vi "Manual-Tester.vi"() -> ()   [LabVIEW 2017]
doc: "Use this template to build a producer/consumer design pattern with events to produce queue items. Use this design pattern instead of the User Interface Event Handler pattern for user interfaces when you want to execute code asynchronously in response to an event without slowing the user interface responsiveness."
uses:
  Events.ctl
  FpgaInterface/FpgaInterface.lvclass
panel:
  out "error out":errorcluster
  in  "error in (no error)":errorcluster
  in  "Write all GPIO":bool
  in  "GPIO #2":u32
  in  "GPIO #1":u32
  out "Elements Remaining":u32
  out "Payload 2":u8[](array[numeric])=[160, 32, 195, 223] format="%.0x"
  out "GPIO #2":u32
  out "GPIO #1":u32
  in  "Payload":u8[](array[numeric])=[160, 32, 195, 223] format="%.0x"
  in  "Read from FIFO #1":bool
  in  "Write to FIFO #1":bool
  out "Status":string
  in  "Read all GPIO":bool
  in  "stop":bool
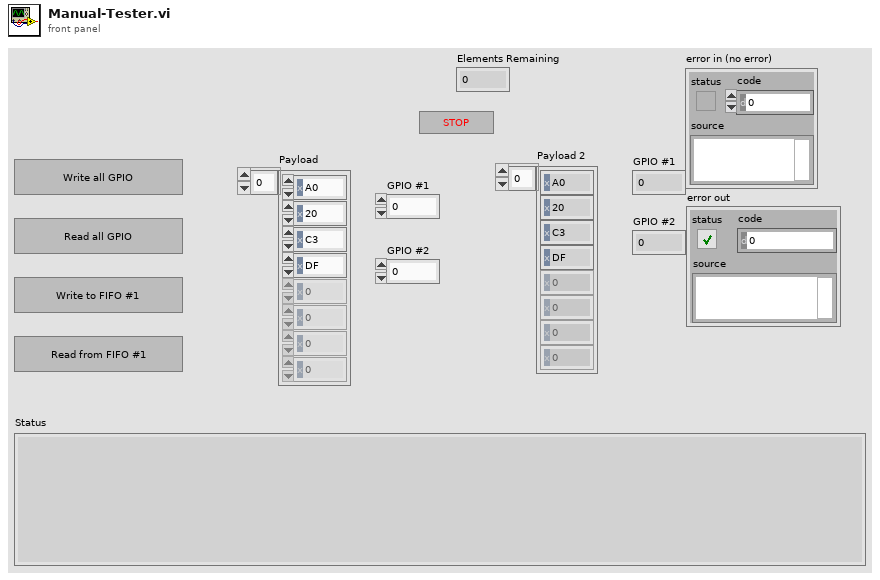
[diagram p1: front panel]
types:
  T1 = typedef "Events.ctl" = enum16{"Open FPGA", "Write to GPIO", "Read all GPIO", "Write to Fifo #1", "Read from Fifo #1", "Close FPGA"}
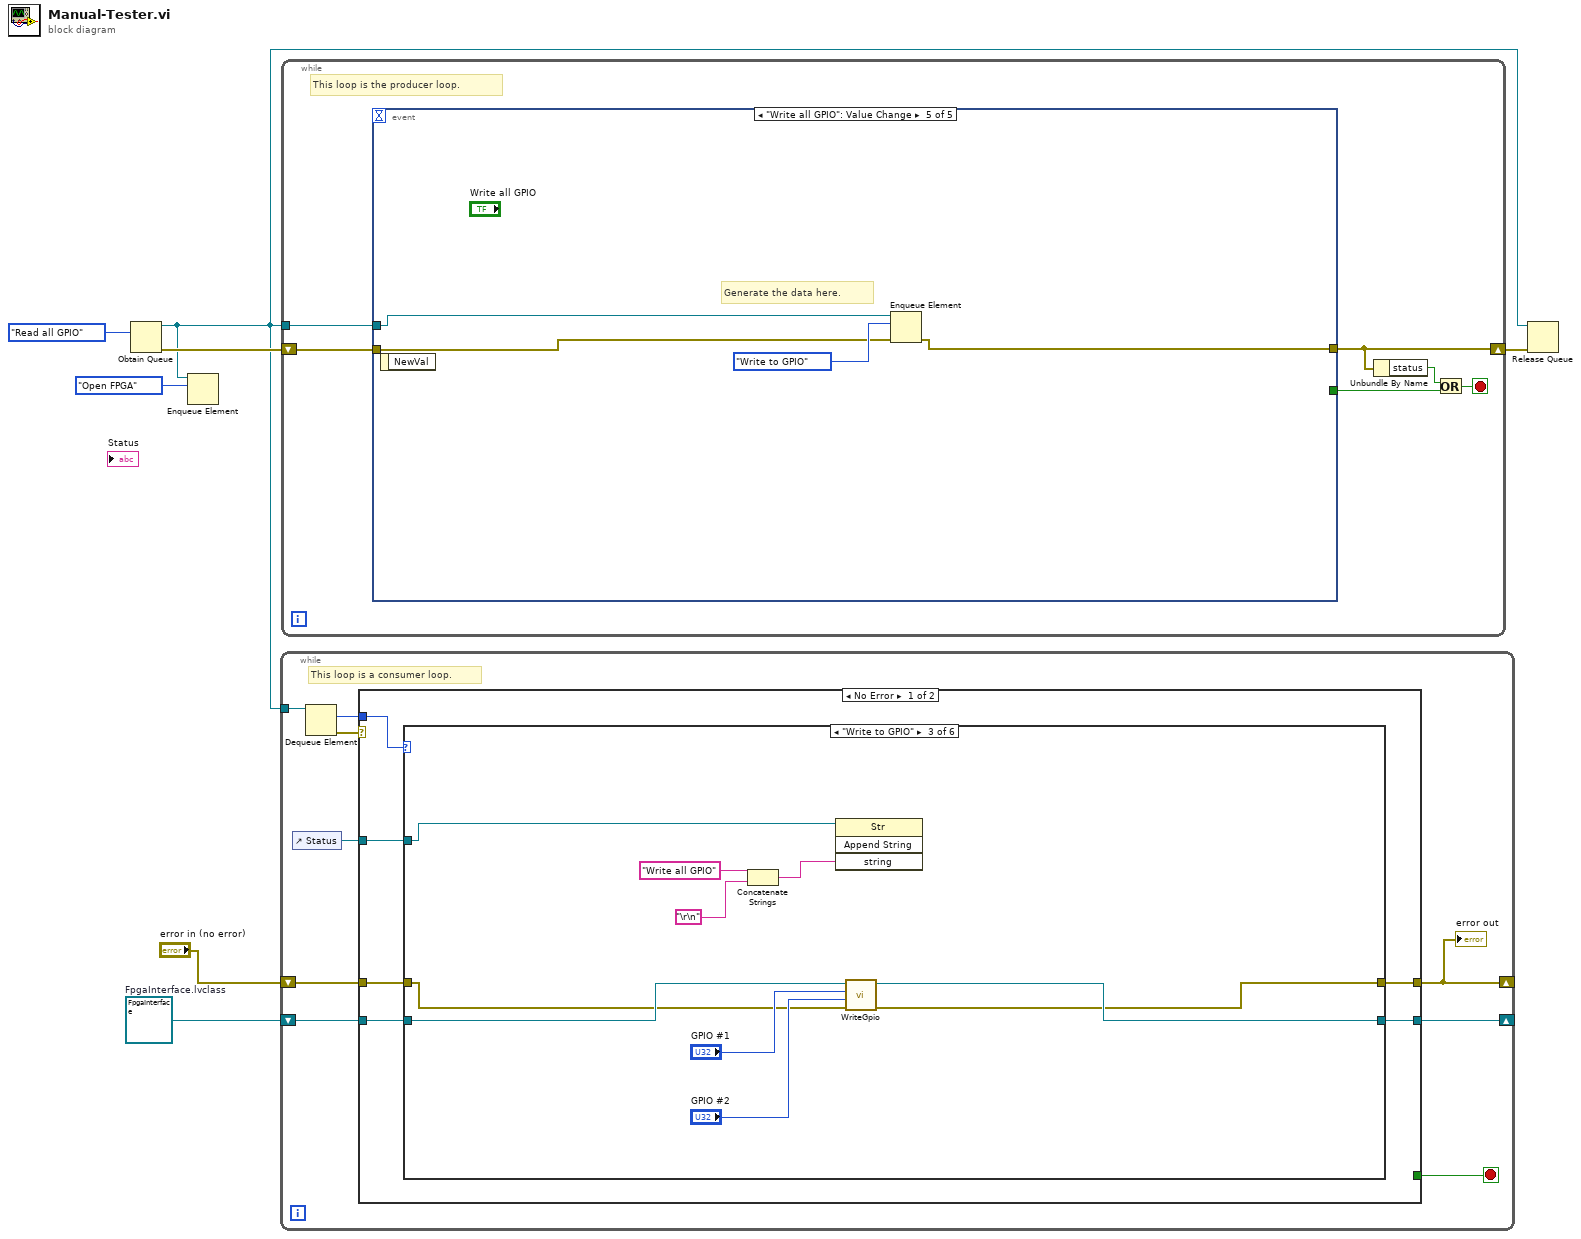
[diagram p0: block diagram]
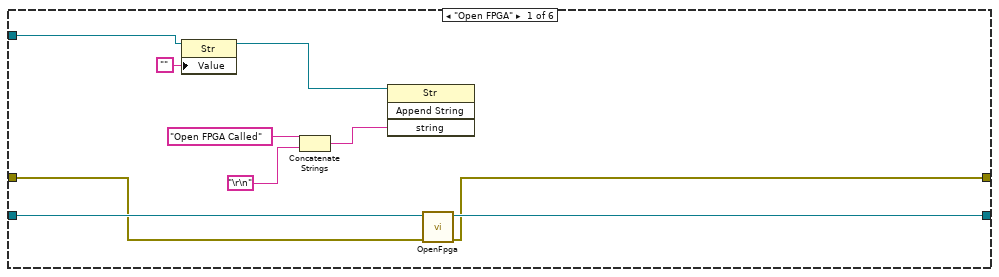
[diagram p2: hidden frame]
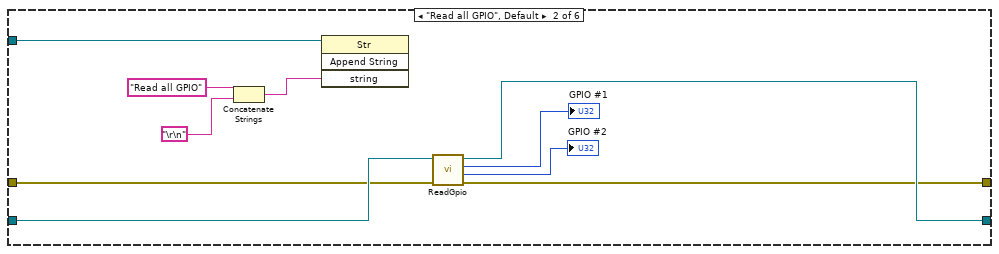
[diagram p3: hidden frame]
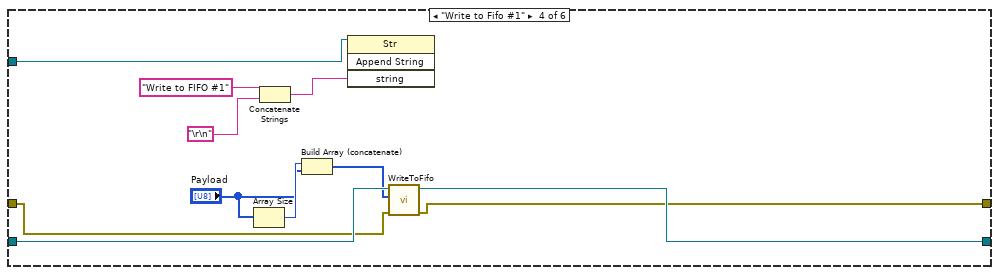
[diagram p4: hidden frame]
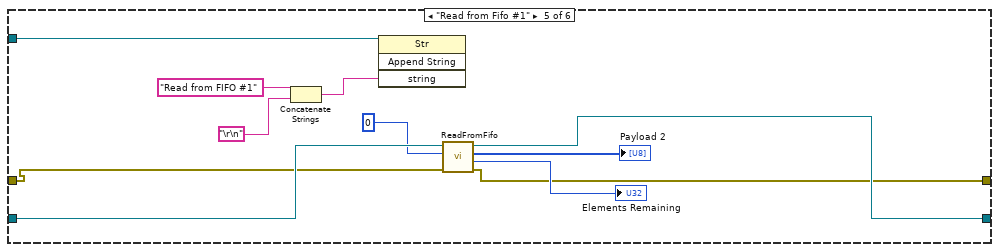
[diagram p5: hidden frame]
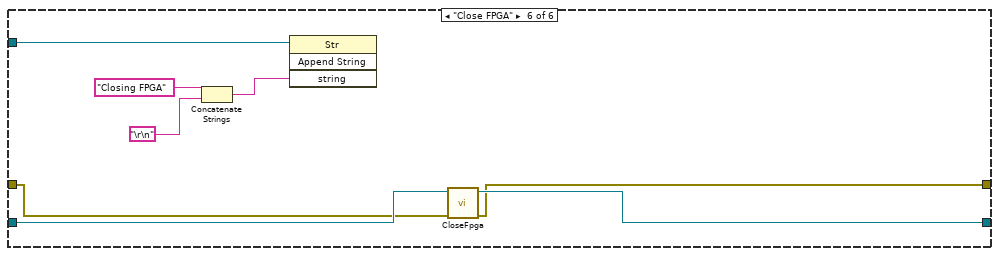
[diagram p6: hidden frame]
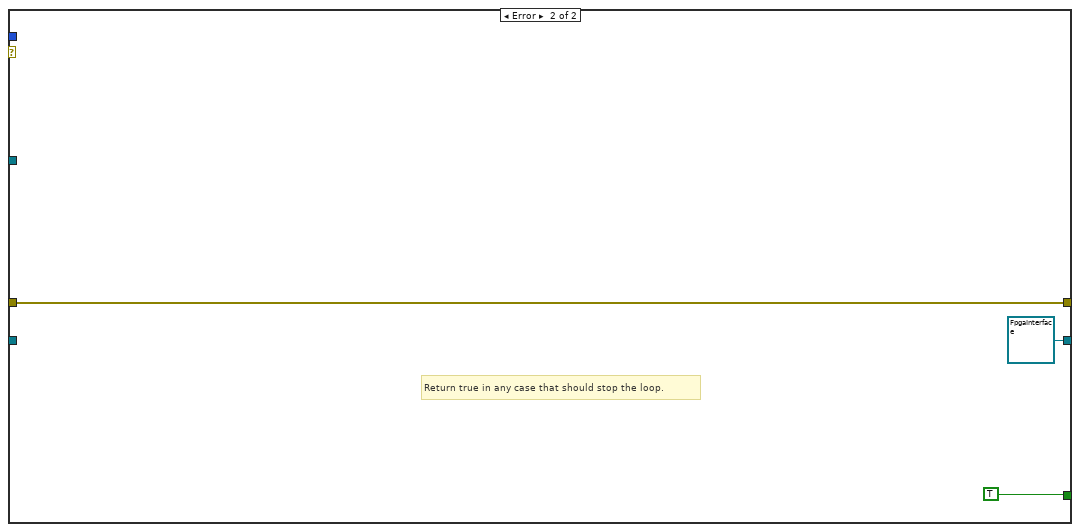
[diagram p7: hidden frame]
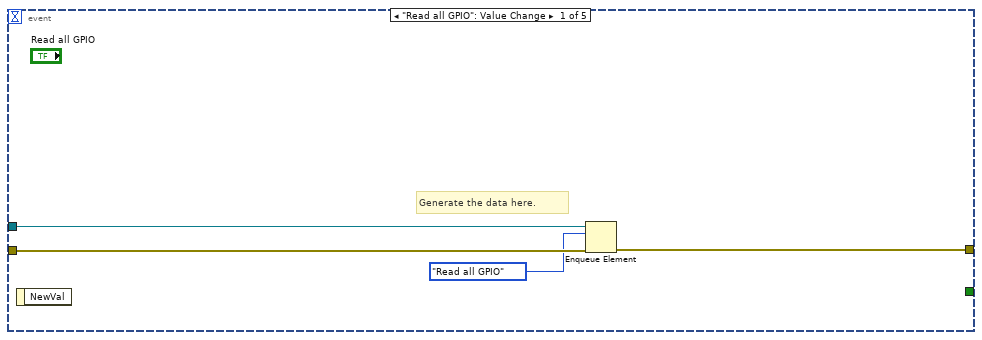
[diagram p8: hidden frame]
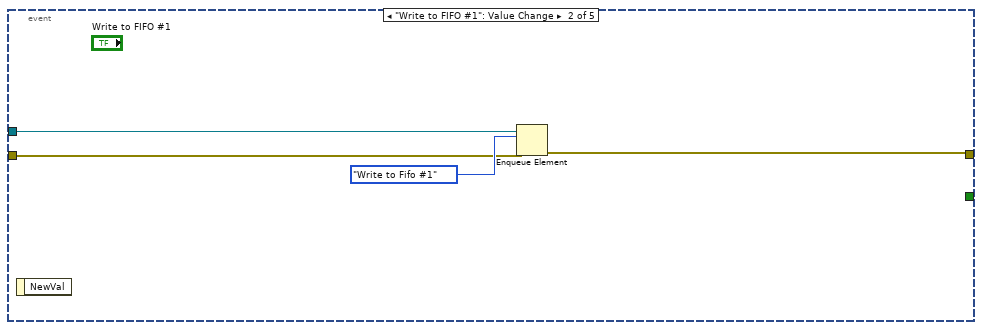
[diagram p9: hidden frame]
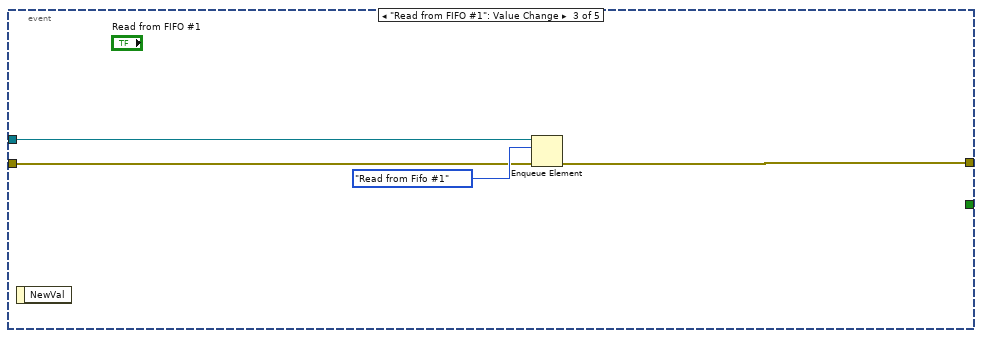
[diagram p10: hidden frame]
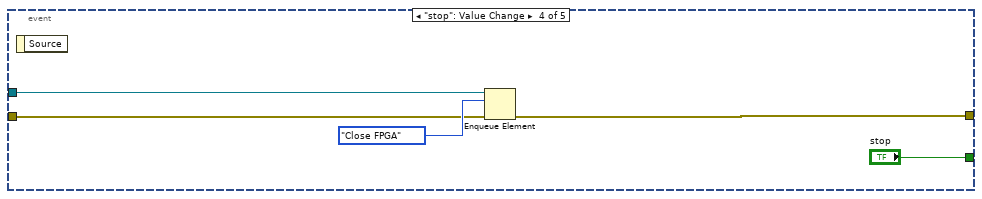
[diagram p11: hidden frame]
diagram:
  w2 = refnum<class "FpgaInterface.lvclass"> refnum  # FpgaInterface.lvclass
  n1 = Obtain Queue(element data type=Events."Read all GPIO" ("Events 2")) -> (queue out=w4:refnum<queue>, error out=w7:errorcluster)  [unwired: 4 in, 1 out]
  n2 = Enqueue Element(queue=w4, element=Events."Open FPGA" ("Events 2")) -> ()  [unwired: 2 in, 3 out]
  n3 = while {
    tunnel: w4 -> [w16]
    shift-right: [w9] -> _
    shift-left: "error in (no error)" -> [w10]
    shift-right: [w8] -> _
    shift-left: w2 -> [w11]
    stop <- w13 stop-if-true
    # "This loop is a consumer loop."
    n4 = control-ref of="Status"() -> (w12:refnum<vi>)
    n5 = Dequeue Element(queue=w16) -> (element=w14:T1, error out=w15:errorcluster)  [unwired: 2 in, 2 out]
    n6 = case shown="No Error" w15 {
      tunnel: w14 -> [w22 _]
      tunnel: [_ TRUE] -> w13
      tunnel: w12 -> [w21 _]
      tunnel: w11 -> [w20 _]
      tunnel: [w19 refnum<class "FpgaInterface.lvclass"> refnum ("FpgaInterface out")] -> w8
      tunnel: w10 -> [w18 w83]
      tunnel: [w17 w83] -> w9
      frame No Error {
        n7 = case shown="\"Write to GPIO\"" w22 {
          tunnel: w21 -> [w27 w39 w49 w60 w71 w79]
          tunnel: w20 -> [w26 w38 w48 w59 w70 w78]
          tunnel: [w25 w35 w45 w58 w67 w77] -> w19
          tunnel: w18 -> [w24 w34 w44 w54 w65 w76]
          tunnel: [w23 w33 w43 w53 w64 w75] -> w17
          frame "Open FPGA" {
            n8 = property class="Str"(reference=w27, "Value"="") -> (reference out=w31:refnum<vi>)  [unwired: 1 in, 1 out]
            n9 = Concatenate Strings("Open FPGA Called" ("string"), "\r\n") -> (w29:string)
            n10 = invoke class="Str" method="Append String"(reference=w31, "string"=w29) -> ()  [unwired: 2 in, 4 out]
            n11 = call-dynamic "OpenFpga.vi"("error in (no error)"=w24, "FpgaInterface in"=w26) -> ("error out"=w23:errorcluster, "FpgaInterface out"=w25:refnum<class "FpgaInterface.lvclass">)  [unwired: 8 in]
          }
          frame "Read all GPIO", Default {
            n12 = Concatenate Strings("Read all GPIO" ("string"), "\r\n") -> (w41:string)
            n13 = invoke class="Str" method="Append String"(reference=w39, "string"=w41) -> ()  [unwired: 2 in, 4 out]
            n14 = call-dynamic "ReadGpio.vi"("error in (no error)"=w34, "FpgaInterface in"=w38) -> ("error out"=w33:errorcluster, "GPIO #2 out"=→"GPIO #2":u32, "GPIO #1 out"=→"GPIO #1":u32, "FpgaInterface out"=w35:refnum<class "FpgaInterface.lvclass">)  [unwired: 6 in]
          }
          frame "Write to GPIO" {
            n15 = Concatenate Strings("Write all GPIO" ("string"), "\r\n") -> (w51:string)
            n16 = invoke class="Str" method="Append String"(reference=w49, "string"=w51) -> ()  [unwired: 2 in, 4 out]
            n17 = call-dynamic "WriteGpio.vi"("error in (no error)"=w44, "GPIO #2 in"="GPIO #2", "GPIO #1 in"="GPIO #1", "FpgaInterface in"=w48) -> ("error out"=w43:errorcluster, "FpgaInterface out"=w45:refnum<class "FpgaInterface.lvclass">)  [unwired: 6 in]
          }
          frame "Write to Fifo #1" {
            n18 = Array Size(array="Payload") -> (size(s)=w57:i32)
            n19 = Concatenate Strings("Write to FIFO #1" ("string"), "\r\n") -> (w62:string)
            n20 = Build Array (concatenate)(w57, "Payload") -> (w55:i32[])
            n21 = invoke class="Str" method="Append String"(reference=w60, "string"=w62) -> ()  [unwired: 2 in, 4 out]
            n22 = call-dynamic "WriteToFifo.vi"("error in (no error)"=w54, "Data"=w55, "FpgaInterface in"=w59) -> ("error out"=w53:errorcluster, "FpgaInterface out"=w58:refnum<class "FpgaInterface.lvclass">)  [unwired: 7 in]
          }
          frame "Read from Fifo #1" {
            n23 = Concatenate Strings("Read from FIFO #1" ("string"), "\r\n") -> (w73:string)
            n24 = invoke class="Str" method="Append String"(reference=w71, "string"=w73) -> ()  [unwired: 2 in, 4 out]
            n25 = call-dynamic "ReadFromFifo.vi"("error in (no error)"=w65, "Number of Elements"=u32 0, "FpgaInterface in"=w70) -> ("error out"=w64:errorcluster, "Elements Remaining"=→"Elements Remaining":u32, "Data"=→"Payload 2":u32[], "FpgaInterface out"=w67:refnum<class "FpgaInterface.lvclass">)  [unwired: 5 in]
          }
          frame "Close FPGA" {
            n26 = Concatenate Strings("Closing FPGA" ("string"), "\r\n") -> (w81:string)
            n27 = invoke class="Str" method="Append String"(reference=w79, "string"=w81) -> ()  [unwired: 2 in, 4 out]
            n28 = call-dynamic "CloseFpga.vi"("error in (no error)"=w76, "FpgaInterface in"=w78) -> ("error out"=w75:errorcluster, "FpgaInterface out"=w77:refnum<class "FpgaInterface.lvclass">)  [unwired: 8 in]
          }
        }
      }
      frame Error {
        # "Return true in any case that should stop the loop."
      }
    }
    "error out" <- w9
  }
  n29 = while {
    shift-right: [w87] -> w6
    shift-left: w7 -> [w90]
    tunnel: w4 -> [w91]
    stop <- w88 stop-if-true
    # "This loop is the producer loop."
    n30 = event shown="[4] \"Write all GPIO\": Value Change" {
      selector: _ -> [_ _ _ _ _]
      dyn-events: _ -> [_ _ _ _ _]
      timeout: _ -> [_ _ _ _ _]
      tunnel: w91 -> [w95 w96 w100 w105 w109]
      tunnel: w90 -> [w94 w98 w102 w106 w110]
      tunnel: [w93 w97 w101 w104 w111] -> w87
      tunnel: [_ _ _ "stop" _] -> w89
      event "Read all GPIO": Value Change {
        # "Generate the data here."
        n31 = event-data() -> ()  [unwired: 1 in, 1 out]
        n32 = Enqueue Element(queue=w95, element=Events."Read all GPIO" ("Events 2"), error in (no error)=w94) -> (error out=w93:errorcluster)  [unwired: 1 in, 2 out]
      }
      event "Write to FIFO #1": Value Change {
        n33 = event-data() -> ()  [unwired: 1 in, 1 out]
        n34 = Enqueue Element(queue=w96, element=Events."Write to Fifo #1" ("Events 2"), error in (no error)=w98) -> (error out=w97:errorcluster)  [unwired: 1 in, 2 out]
      }
      event "Read from FIFO #1": Value Change {
        n35 = event-data() -> ()  [unwired: 1 in, 1 out]
        n36 = Enqueue Element(queue=w100, element=Events."Read from Fifo #1" ("Events 2"), error in (no error)=w102) -> (error out=w101:errorcluster)  [unwired: 1 in, 2 out]
      }
      event "stop": Value Change {
        n37 = event-data() -> ()  [unwired: 1 in, 1 out]
        n38 = Enqueue Element(queue=w105, element=Events."Close FPGA" ("Events 2"), error in (no error)=w106) -> (error out=w104:errorcluster)  [unwired: 1 in, 2 out]
      }
      event "Write all GPIO": Value Change {
        # "Generate the data here."
        n39 = event-data() -> ()  [unwired: 1 in, 1 out]
        n40 = Enqueue Element(queue=w109, element=Events."Write to GPIO" ("Events 2"), error in (no error)=w110) -> (error out=w111:errorcluster)  [unwired: 1 in, 2 out]
      }
    }
    n41 = Unbundle By Name(w87) -> ("status"=w86:bool)
    n42 = Or(x=w86, y=w89) -> (x .or. y?=w88:bool)
  }
  n43 = Release Queue(queue=w4, error in (no error)=w6) -> ()  [unwired: 1 in, 3 out]
